vi "Muon direction to polar coordinate.vi"() -> ()   [LabVIEW 2016]
uses:
  Typedefs/Coincidence.ctl
  <vilib>/Analysis/coordinate.llb/3D Coordinate Conversion (Scalar).vi
  <vilib>/gmath/interp.llb/Interpolate 2D (2d X,Y).vi
  <vilib>/Analysis/NI_AALPro.lvlib
  <vilib>/gmath/NI_Gmath.lvlib
panel:
  in  "Good single track hits":cluster{"CRT-wide coincs":T1[]}[](array[cluster])
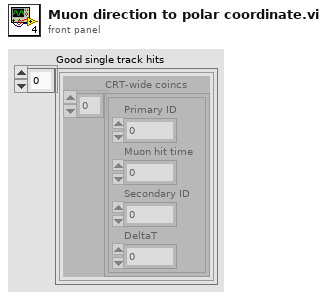
[diagram p1: front panel]
types:
  T1 = typedef "Coincidence.ctl" = cluster{"Primary ID":i8, "Muon hit time":u64, "Secondary ID":i8, "DeltaT":i32}
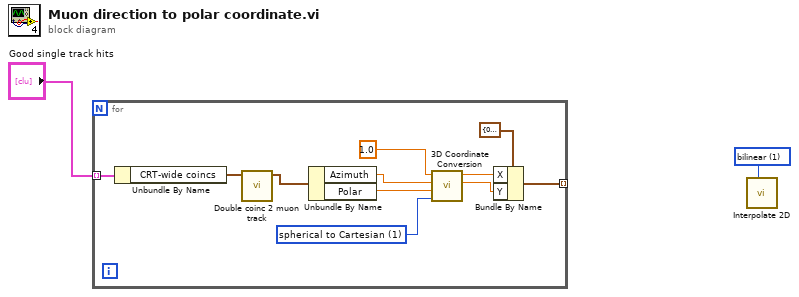
[diagram p0: block diagram]
diagram:
  w1 = 1 items=["nearest", "bilinear", "bicubic", "bicubic spline"] ("method")
  n1 = for {
    tunnel: "Good single track hits" -> [w13] mode=indexing
    tunnel: [w3] -> _ mode=indexing
    w10 = u16 1 items=["Cartesian to spherical", "spherical to Cartesian", "Cartesian to cylindrical", "cylindrical to Cartesian", "spherical to cylindrical", "cylindrical to spherical"] ("conversion type")
    n2 = Unbundle By Name(w13) -> ("CRT-wide coincs"=w12:T1[])
    n3 = call "Double coinc 2 muon track.vi"("Array of two hits"=w12) -> ("Muon track"=w11:cluster{"Azimuth":dbl, "Polar":dbl})  [unwired: 10 in]
    n4 = Unbundle By Name(w11) -> ("Azimuth"=w8:dbl, "Polar"=w7:dbl)
    n5 = call-poly <vilib>:"3D Coordinate Conversion.vi"("conversion type"=w10, "axis 3"=w7, "axis 2"=w8, "axis 1"=1.0) -> ("axis 2 out"=w4:dbl, "axis 1 out"=w5:dbl)  [unwired: 4 in, 2 out]
    n6 = Bundle By Name(cluster=cluster{"X":dbl, "Y":dbl} {"X"=0.0, "Y"=0.0}, "X"=w5, "Y"=w4) -> (w3:cluster{"X":dbl, "Y":dbl})
  }
  n7 = call-poly <vilib>:"Interpolate 2D.vi"("method"=w1) -> ()  [unwired: 7 in, 4 out]
